vi "test Passes If Arrays Are Equal.vi"(8 "error in (no error)":errorcluster, 11 "TestCase in":refnum<class "Pass If Equal 1D Array (Boolean) Test Case.lvclass">) -> (0 "error out":errorcluster, 3 "TestCase out":refnum<class "Pass If Equal 1D Array (Boolean) Test Case.lvclass">)   [LabVIEW 2015, in "Pass If Equal 1D Array (Boolean) Test Case.lvclass"]
uses:
  Pass If Equal 1D Array (Boolean) Test Case.lvclass
  <vilib>/addons/_JKI Toolkits/VI Tester/TestCase.llb/TestCase.lvclass
  VITAC.lvlib
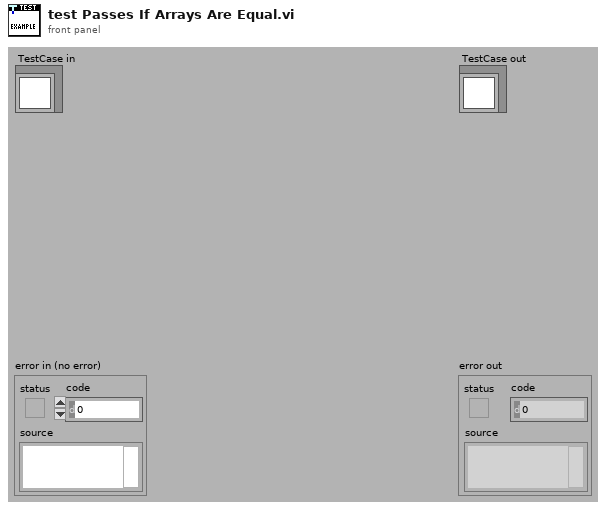
[diagram p1: front panel]
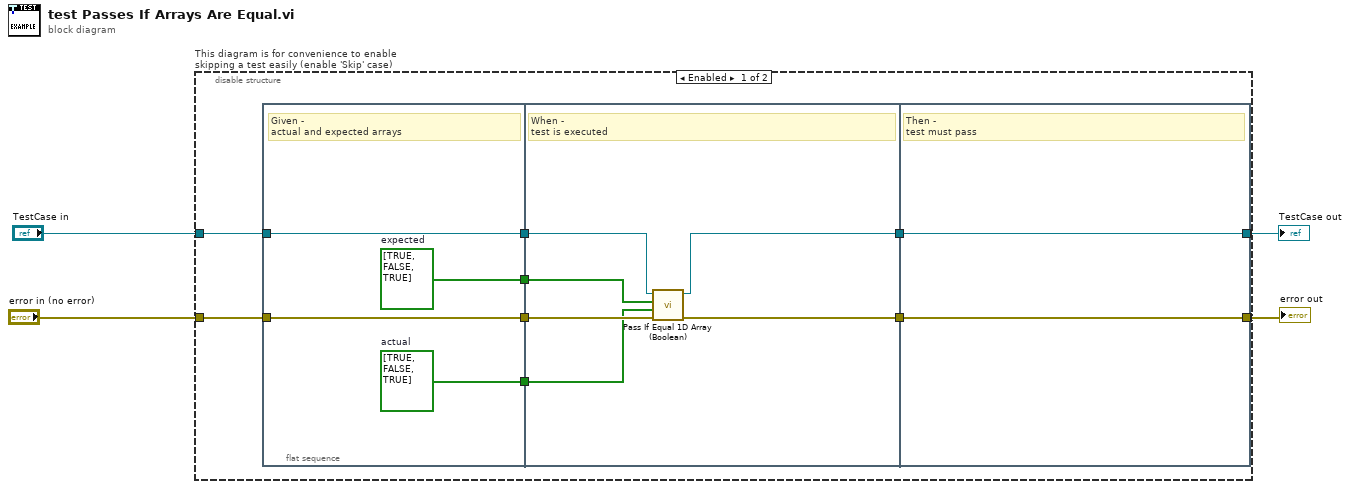
[diagram p0: block diagram]
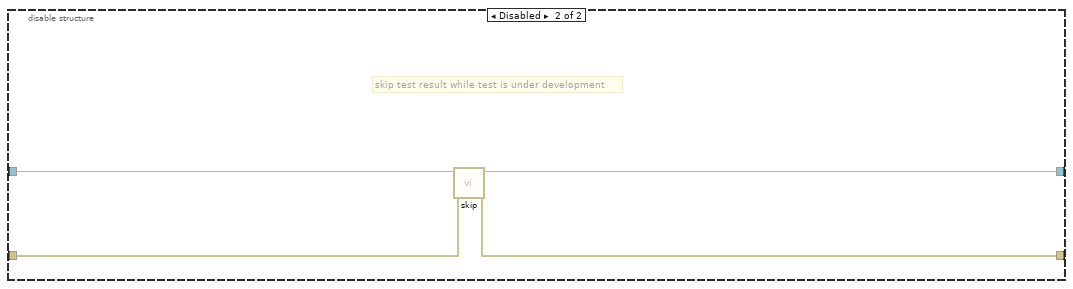
[diagram p2: hidden frame]
diagram:
  n1 = disable-structure "This diagram is for convenience to enable skipping a test easily (enable 'Skip' case)" shown="Enabled" {
    disable-tunnel: "TestCase in" -> [w9 w30]
    disable-tunnel: [w8 w28] -> w1
    disable-tunnel: [w12 w29] -> w3
    disable-tunnel: "error in (no error)" -> [w13 w27]
    frame Enabled {
      n2 = flat-sequence {
        tunnel: [w18] -> w14
        tunnel: w13 -> [w18]
        tunnel: [w17] -> w10
        tunnel: w9 -> [w17]
        tunnel: [w16] -> w6
        tunnel: [w15] -> w5
        tunnel: w14 -> [w24]
        tunnel: [w23] -> w11
        tunnel: w10 -> [w22]
        tunnel: [w21] -> w7
        tunnel: w6 -> [w20]
        tunnel: w5 -> [w19]
        tunnel: [w26] -> w12
        tunnel: w11 -> [w26]
        tunnel: [w25] -> w8
        tunnel: w7 -> [w25]
        frame #0 {
          w16 = bool[] [TRUE, FALSE, TRUE]  # expected
          w15 = bool[] [TRUE, FALSE, TRUE]  # actual
          # "Given - \nactual and expected arrays"
        }
        frame #1 {
          # "When - \ntest is executed"
          n3 = call "Pass If Equal 1D Array (Boolean).vi"("error in (no error)"=w24, "actual"=w19, "expected"=w20, "TestCase in"=w22) -> ("error out"=w23:errorcluster, "TestCase out"=w21:refnum<class "Pass If Equal 1D Array (Boolean) Test Case.lvclass">)  [unwired: 6 in]
        }
        frame #2 {
          # "Then - \ntest must pass"
        }
      }
    }
    frame Disabled {
      # "skip test result while test is under development"
      n4 = call <vilib>:"skip.vi"("error in (no error)"=w27, "TestCase in"=w30) -> ("error out"=w29:errorcluster, "TestCase out"=w28:refnum<class "Pass If Equal 1D Array (Boolean) Test Case.lvclass">)  [unwired: 8 in]
    }
  }
  "error out" <- w3
  "TestCase out" <- w1
